vi "latency.vi"(11 "input":dbl[](array[numeric])) -> (2 "N1_latency":dbl, 3 "P3_latency":dbl)   [LabVIEW 2014]
uses:
  <vilib>/Analysis/baseanly.llb/Mean (DBL).vi
  <vilib>/Analysis/NI_AALBase.lvlib
panel:
  in  "rate":dbl=20.0 caption="Rate" format="%0.2f"
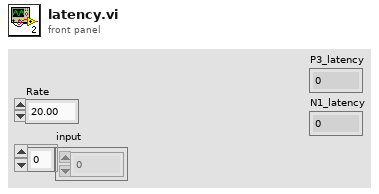
[diagram p1: front panel]
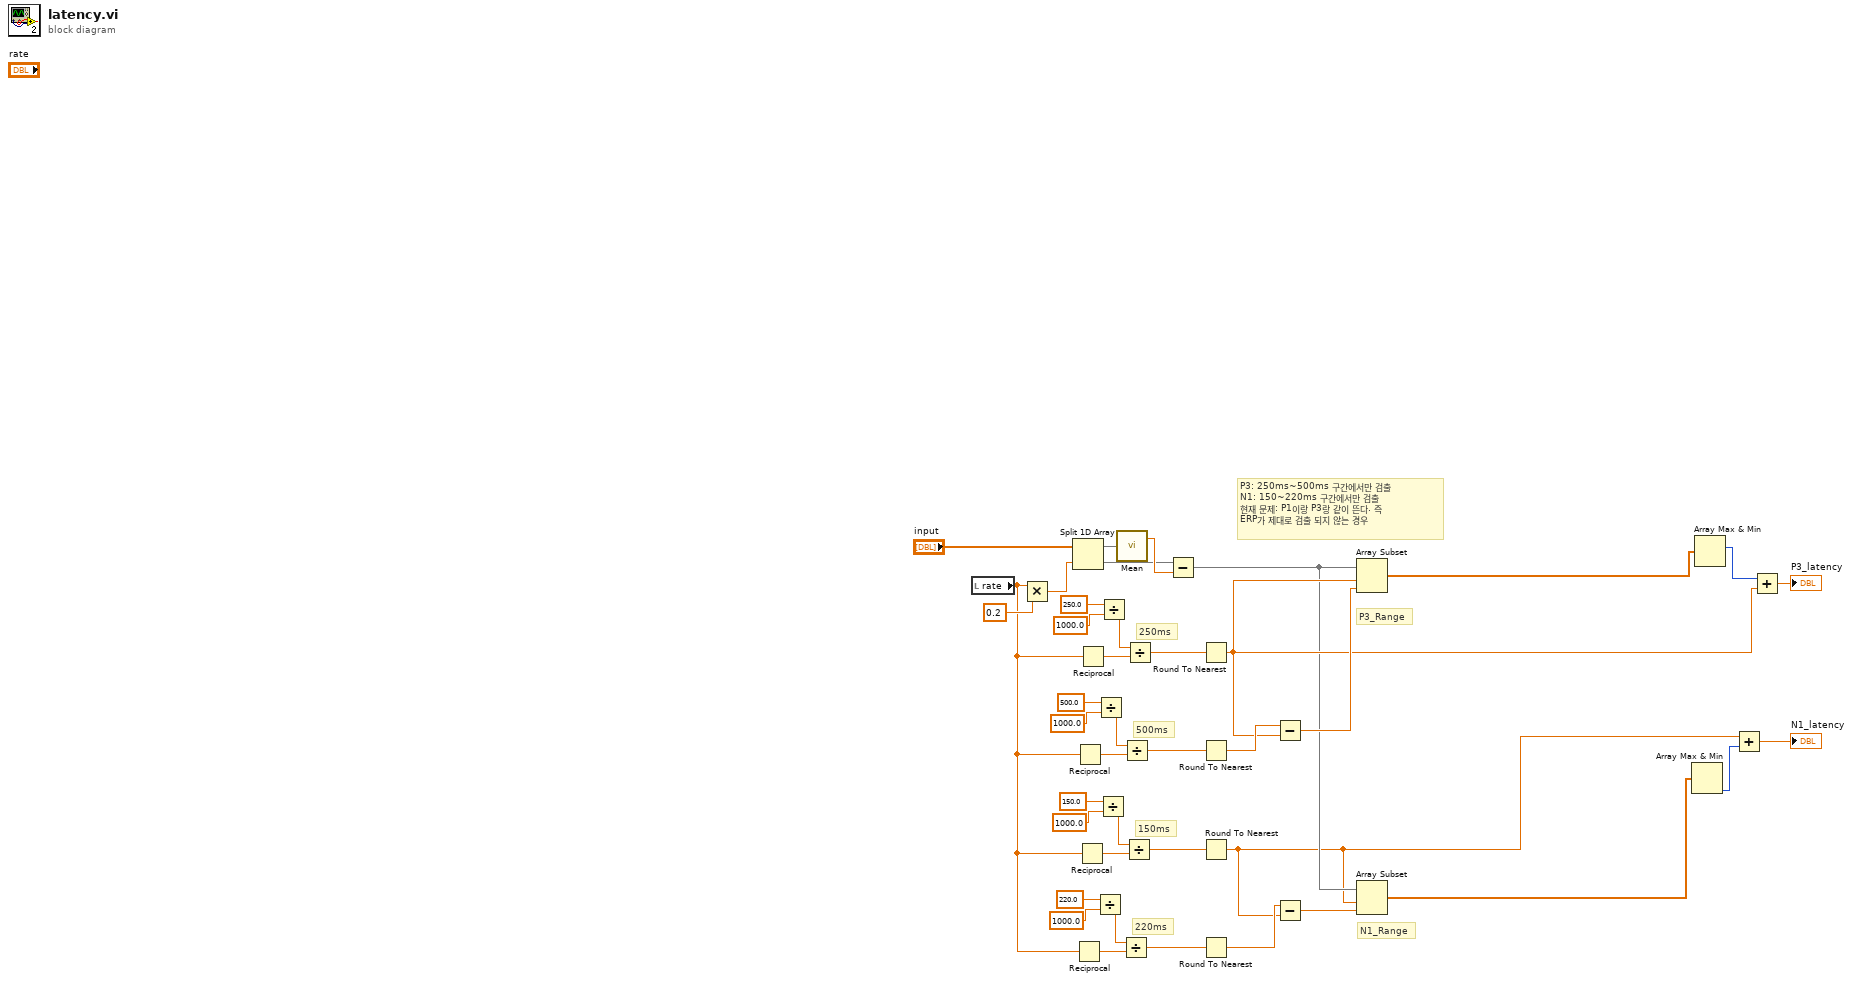
[diagram p0: block diagram]
diagram:
  # "N1_Range"
  # "P3_Range"
  # "220ms"
  # "150ms"
  # "500ms"
  # "250ms"
  # "P3: 250ms~500ms 구간에서만 검출\nN1: 150~220ms 구간에서만 검출\n현재 문제: P1이랑 P3랑 같이 뜬다. 즉\nERP가 제대로 검출 되지 않는 경우"
  n1 = local read "rate"() -> (w17:dbl)
  n2 = Multiply(x=w17, y=0.2) -> (x*y=w39:dbl)
  n3 = Split 1D Array(array="input", index=w39) -> (first subarray=w38:dbl[], second subarray=w36:dbl[])
  n4 = Reciprocal(x=w17) -> (1/x=w21:dbl)
  n5 = Reciprocal(x=w17) -> (1/x=w29:dbl)
  n6 = Reciprocal(x=w17) -> (1/x=w25:dbl)
  n7 = Reciprocal(x=w17) -> (1/x=w33:dbl)
  n8 = Divide(x=220.0, y=1000.0) -> (x/y=w18:dbl)
  n9 = Divide(x=500.0, y=1000.0) -> (x/y=w26:dbl)
  n10 = Divide(x=150.0, y=1000.0) -> (x/y=w22:dbl)
  n11 = Divide(x=250.0, y=1000.0) -> (x/y=w30:dbl)
  n12 = call-poly <vilib>:"Mean.vi"("X"=w38) -> ("mean"=w37:dbl)  [unwired: 1 out]
  n13 = Divide(x=w18, y=w21) -> (x/y=w13:dbl)
  n14 = Divide(x=w26, y=w29) -> (x/y=w15:dbl)
  n15 = Divide(x=w22, y=w25) -> (x/y=w14:dbl)
  n16 = Divide(x=w30, y=w33) -> (x/y=w16:dbl)
  n17 = Subtract(x=w36, y=w37) -> (x-y=w6:dbl[])
  n18 = Round To Nearest(number=w16) -> (nearest integer value=w10:dbl)
  n19 = Round To Nearest(number=w15) -> (nearest integer value=w12:dbl)
  n20 = Round To Nearest(number=w14) -> (nearest integer value=w4:dbl)
  n21 = Round To Nearest(number=w13) -> (nearest integer value=w7:dbl)
  n22 = Subtract(x=w12, y=w10) -> (x-y=w11:dbl)
  n23 = Subtract(x=w7, y=w4) -> (x-y=w8:dbl)
  n24 = Array Subset(array=w6, index=w10, length=w11) -> (w9:dbl[])
  n25 = Array Subset(array=w6, index=w4, length=w8) -> (w5:dbl[])
  n26 = Array Max & Min(array=w5) -> (min index (indices)=w35:i32)  [unwired: 3 out]
  n27 = Array Max & Min(array=w9) -> (max index (indices)=w34:i32)  [unwired: 3 out]
  n28 = Add(x=w4, y=w35) -> (x+y=→"N1_latency":dbl)
  n29 = Add(x=w34, y=w10) -> (x+y=→"P3_latency":dbl)
